vi "DSF Configuration File to Cluster.vi"(8 "error in (no error)":errorcluster, 11 "dsf configuration file path":path) -> (0 "error out":errorcluster, 2 "framework configuration out":T1, 3 "dsf configuration file path dup":path)   [LabVIEW 2017, in "DSF Core.lvlib"]
uses:
  DSF Core.lvlib
  DSF Configuration API/Public/Controls/DSF Engine Framework Configuration.ctl
  DSF Configuration API/Public/Controls/DSF Engine Plugin Configuration.ctl
  DSF Configuration API/Public/Controls/DSF Timing Info.ctl
  DSF Configuration API/Public/Controls/DSF Engine Plugin Thread Configuration.ctl
  DSF Configuration API/Public/Controls/DSF Settings Info.ctl
  DSF Configuration API/Public/Controls/DSF Engine Transfer Group Configuration.ctl
  DSF Configuration API/Public/Controls/DSF Direction.ctl
  DSF Configuration API/Public/Controls/DSF Engine Transfer Configuration.ctl
  DSF Configuration API/Public/Controls/DSF Byte Order.ctl
  DSF Configuration API/Public/Controls/DSF Engine Channel Configuration.ctl
  DSF Configuration API/Public/Controls/DSF Channel Buffer Descriptor.ctl
  DSF Configuration API/Public/Controls/DSF Data Type.ctl
  DSF Configuration API/Public/Read All Item IDs/Read All Plugin IDs.vi
  DSF Configuration API/Public/Read Item/Read Plugin.vi
  DSF Configuration API/Public/Read Item/Read Settings.vi
  DSF Configuration API/Public/Read Item/Read Group.vi
  DSF Configuration API/Public/Read Item/Read Transfer.vi
  DSF Configuration API/Public/Read Item/Read Channel.vi
  DSF Configuration API/Configuration Session.lvclass
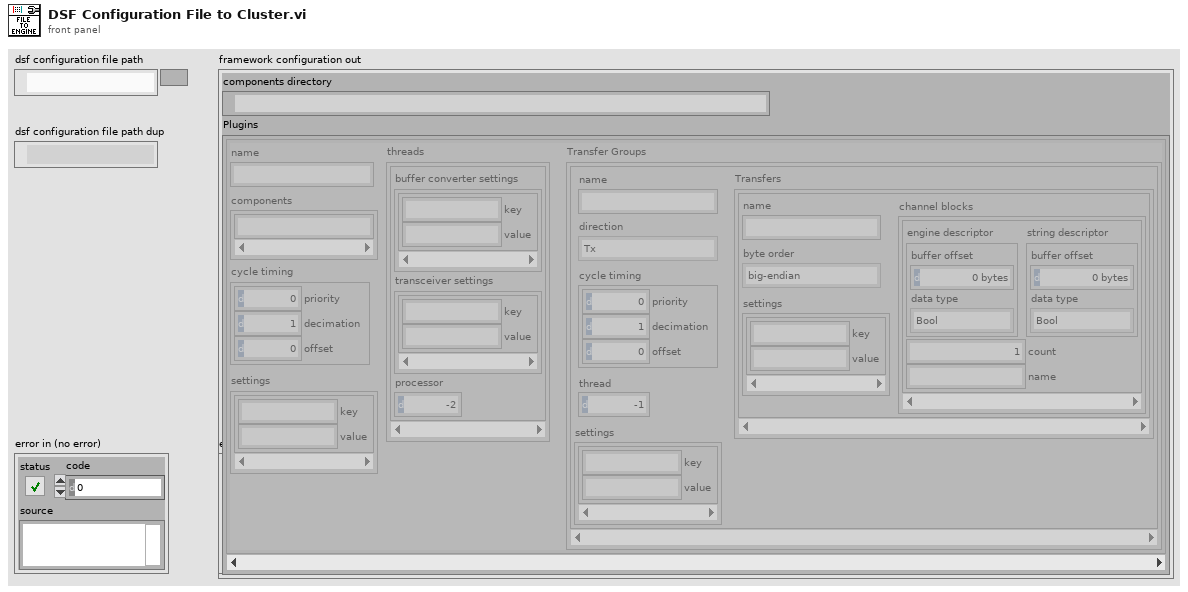
[diagram p1: front panel]
types:
  T1 = typedef "DSF Core.lvlib/DSF Engine Framework Configuration.ctl" = cluster{"components directory":path, "Plugins":T2[]}
  T2 = typedef "DSF Core.lvlib/DSF Engine Plugin Configuration.ctl" = cluster{"name":string, "components":string[], "cycle timing":T3, "threads":T4[], "Transfer Groups":T6[], "settings":T5}
  T3 = typedef "DSF Core.lvlib/DSF Timing Info.ctl" = cluster{"priority":u64, "decimation":u64, "offset":u64}
  T4 = typedef "DSF Core.lvlib/DSF Engine Plugin Thread Configuration.ctl" = cluster{"buffer converter settings":T5, "transceiver settings":T5, "processor":i32}
  T5 = typedef "DSF Core.lvlib/DSF Settings Info.ctl" = cluster{"key":string, "value":string}[]
  T6 = typedef "DSF Core.lvlib/DSF Engine Transfer Group Configuration.ctl" = cluster{"name":string, "direction":T7, "cycle timing":T3, "thread":i32, "settings":T5, "Transfers":T8[]}
  T7 = typedef "DSF Core.lvlib/DSF Direction.ctl" = enum8{"Tx", "Rx"}
  T8 = typedef "DSF Core.lvlib/DSF Engine Transfer Configuration.ctl" = cluster{"name":string, "byte order":T9, "channel blocks":T10[], "settings":T5}
  T9 = typedef "DSF Core.lvlib/DSF Byte Order.ctl" = enum8{"big-endian", "little-endian"}
  T10 = typedef "DSF Core.lvlib/DSF Engine Channel Configuration.ctl" = cluster{"engine descriptor":T11, "string descriptor":T11, "count":u64, "name":string}
  T11 = typedef "DSF Core.lvlib/DSF Channel Buffer Descriptor.ctl" = cluster{"buffer offset":u64, "data type":T12}
  T12 = typedef "DSF Core.lvlib/DSF Data Type.ctl" = enum8{"Bool", "SGL", "DBL", "I8", "I16", "I32", "I64", "U8", "U16", "U32", "U64"}
  T13 = typedef "DSF Core.lvlib/DSF Plugin Info.ctl" = cluster{"components":string[], "timing":T3, "group ids":string[], "settings id":string, "threads":T4[]}
  T14 = typedef "DSF Core.lvlib/DSF Group Info.ctl" = cluster{"direction":T7, "timing":T3, "transfer ids":string[], "settings id":string, "thread":i32}
  T15 = typedef "DSF Core.lvlib/DSF Transfer Info.ctl" = cluster{"byte order":T9, "channel ids":string[], "settings id":string}
  T16 = typedef "DSF Core.lvlib/DSF Channel Info.ctl" = cluster{"count":u64, "string buffer offset":u64, "engine buffer offset":u64, "string data type":T12, "engine data type":T12, "settings id":string}
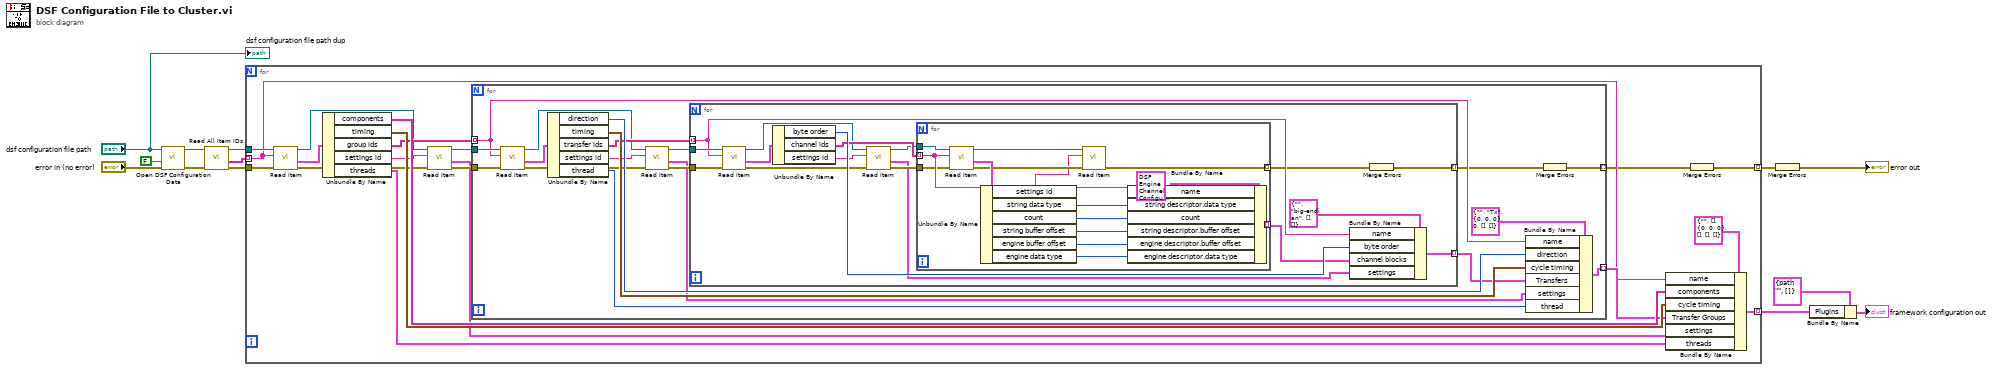
[diagram p0: block diagram]
diagram:
  n1 = call "Open DSF Configuration Data.vi"("error in (no error)"="error in (no error)", "replace if found? (F)"=FALSE ("create file if necessary (T)"), "dsf configuration file path"="dsf configuration file path") -> ("error out"=w4:errorcluster, "Configuration Session"=w5:refnum<class "Configuration Session.lvclass">)  [unwired: 4 in, 3 out]
  n2 = call-poly "Read All Item IDs.vi"("error in (no error)"=w4, "Configuration Session in"=w5) -> ("error out"=w10:errorcluster, "Plugin IDs"=w12:string[], "Configuration Session out"=w11:refnum<class "Configuration Session.lvclass">)  [unwired: 7 in]
  n3 = for {
    tunnel: w12 -> [w24] mode=indexing
    tunnel: w11 -> [w31]
    tunnel: [w27] -> w6 mode=indexing
    tunnel: w10 -> [w19]
    tunnel: [w16] -> w9 mode=indexing
    n4 = call-poly "Read Item.vi"("error in (no error)"=w19, "Plugin ID"=w24, "Configuration Session in"=w31) -> ("error out"=w20:errorcluster, "value"=w30:T13, "Configuration Session out"=w23:refnum<class "Configuration Session.lvclass">)  [unwired: 5 in, 1 out]
    n5 = Unbundle By Name(w30) -> ("components"=w29:string[], "timing"=w28:T3, "group ids"=w26:string[], "settings id"=w21:string, "threads"=w15:T4[])
    n6 = call-poly "Read Item.vi"("error in (no error)"=w20, "Settings ID"=w21, "Configuration Session in"=w23) -> ("error out"=w18:errorcluster, "value"=w14:T5, "Configuration Session out"=w22:refnum<class "Configuration Session.lvclass">)  [unwired: 5 in, 1 out]
    n7 = for {
      tunnel: w22 -> [w51]
      tunnel: w26 -> [w48] mode=indexing
      tunnel: [w45] -> w25 mode=indexing
      tunnel: w18 -> [w42]
      tunnel: [w34] -> w17 mode=indexing
      n8 = call-poly "Read Item.vi"("error in (no error)"=w42, "Group ID"=w48, "Configuration Session in"=w51) -> ("error out"=w38:errorcluster, "value"=w49:T14, "Configuration Session out"=w41:refnum<class "Configuration Session.lvclass">)  [unwired: 5 in, 1 out]
      n9 = Unbundle By Name(w49) -> ("direction"=w47:T7, "timing"=w46:T3, "transfer ids"=w44:string[], "settings id"=w39:string, "thread"=w33:i32)
      n10 = call-poly "Read Item.vi"("error in (no error)"=w38, "Settings ID"=w39, "Configuration Session in"=w41) -> ("error out"=w37:errorcluster, "value"=w36:T5, "Configuration Session out"=w40:refnum<class "Configuration Session.lvclass">)  [unwired: 5 in, 1 out]
      n11 = for {
        tunnel: w44 -> [w61] mode=indexing
        tunnel: w40 -> [w68]
        tunnel: [w65] -> w43 mode=indexing
        tunnel: w37 -> [w60]
        tunnel: [w53] -> w35 mode=indexing
        n12 = call-poly "Read Item.vi"("error in (no error)"=w60, "Transfer ID"=w61, "Configuration Session in"=w68) -> ("error out"=w58:errorcluster, "value"=w67:T15, "Configuration Session out"=w62:refnum<class "Configuration Session.lvclass">)  [unwired: 5 in, 1 out]
        n13 = Unbundle By Name(w67) -> ("byte order"=w66:T9, "channel ids"=w63:string[], "settings id"=w57:string)
        n14 = call-poly "Read Item.vi"("error in (no error)"=w58, "Settings ID"=w57, "Configuration Session in"=w62) -> ("error out"=w56:errorcluster, "value"=w55:T5, "Configuration Session out"=w59:refnum<class "Configuration Session.lvclass">)  [unwired: 5 in, 1 out]
        n15 = for {
          tunnel: [w83] -> w64 mode=indexing
          tunnel: w63 -> [w81] mode=indexing
          tunnel: w59 -> [w82]
          tunnel: w56 -> [w76]
          tunnel: [w73] -> w54 mode=indexing
          n16 = call-poly "Read Item.vi"("error in (no error)"=w76, "Channel ID"=w81, "Configuration Session in"=w82) -> ("error out"=w74:errorcluster, "value"=w80:T16, "Configuration Session out"=w75:refnum<class "Configuration Session.lvclass">)  [unwired: 5 in, 1 out]
          n17 = Unbundle By Name(w80) -> ("settings id"=w71:string, "string data type"=w79:T12, "count"=w78:u64, "string buffer offset"=w77:u64, "engine buffer offset"=w70:u64, "engine data type"=w69:T12)
          n18 = call-poly "Read Item.vi"("error in (no error)"=w74, "Settings ID"=w71, "Configuration Session in"=w75) -> ("error out"=w73:errorcluster)  [unwired: 5 in, 3 out]
          n19 = Bundle By Name(cluster=T10 {"engine descriptor"={"buffer offset"=0, "data type"=enum."Bool"}, "string descriptor"={"buffer offset"=0, "data type"=enum."Bool"}, "count"=0, "name"=""} ("channel configurations"), "name"=w81, "string descriptor.data type"=w79, "count"=w78, "string descriptor.buffer offset"=w77, "engine descriptor.buffer offset"=w70, "engine descriptor.data type"=w69) -> (w83:T10)
        }
        n20 = Bundle By Name(cluster=T8 {"name"="", "byte order"=enum."big-endian", "channel blocks"=[], "settings"=[]} ("Transfer Configuration"), "name"=w61, "byte order"=w66, "channel blocks"=w64, "settings"=w55) -> (w65:T8)
        n21 = Merge Errors(w54) -> (w53:errorcluster)
      }
      n22 = Bundle By Name(cluster=T6 {"name"="", "direction"=enum."Tx", "cycle timing"={"priority"=0, "decimation"=0, "offset"=0}, "thread"=0, "settings"=[], "Transfers"=[]} ("Transfer Group Configuration"), "name"=w48, "direction"=w47, "cycle timing"=w46, "Transfers"=w43, "settings"=w36, "thread"=w33) -> (w45:T6)
      n23 = Merge Errors(w35) -> (w34:errorcluster)
    }
    n24 = Bundle By Name(cluster=T2 {"name"="", "components"=[], "cycle timing"={"priority"=0, "decimation"=0, "offset"=0}, "threads"=[], "Transfer Groups"=[], "settings"=[]} ("Plugin Configuration"), "name"=w24, "components"=w29, "cycle timing"=w28, "Transfer Groups"=w25, "settings"=w14, "threads"=w15) -> (w27:T2)
    n25 = Merge Errors(w17) -> (w16:errorcluster)
  }
  n26 = Merge Errors(w9) -> (→"error out":errorcluster)
  n27 = Bundle By Name(cluster=T1 {"components directory"=path "", "Plugins"=[]} ("Framework Config (JSON)"), "Plugins"=w6) -> (→"framework configuration out":T1)
  "dsf configuration file path dup" <- "dsf configuration file path"
